vi "i.vi"(1 "start":bool) -> (0 "i":i32)   [LabVIEW 2019]
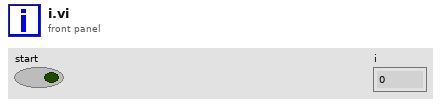
[diagram p1: front panel]
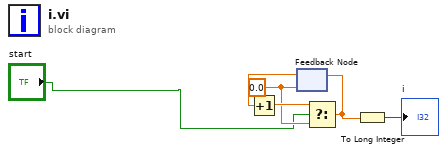
[diagram p0: block diagram]
diagram:
  w2 = 0.0
  n1 = feedback #1(w2) -> (w6:dbl)
  n2 = Increment(x=w6) -> (x+1=w3:dbl)
  n3 = Select(t=w3, s="start", f=w2) -> (s? t:f=w5:dbl)
  n4 = feedback-in #1(w5) -> ()
  n5 = To Long Integer(number=w5) -> (32bit integer=→"i":i32)
